vi "Neighbor.vi"(7 "Goal":T1, 10 "Dir":T2, 11 "Position":T1) -> (3 "Neighbor":T1, 5 "In Bounds":bool)   [LabVIEW 2020]
uses:
  Position.ctl
  Dir.ctl
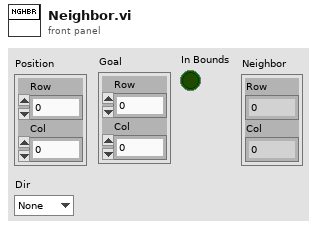
[diagram p1: front panel]
types:
  T1 = typedef "Position.ctl" = cluster{"Row":i32, "Col":i32}
  T2 = typedef "Dir.ctl" = enum16{"None", "Up", "Left", "Down", "Right"}
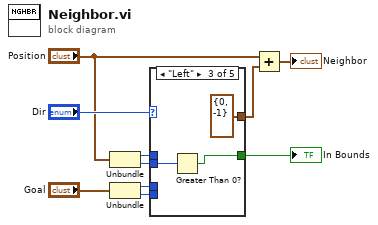
[diagram p0: block diagram]
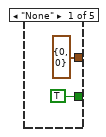
[diagram p2: hidden frame]
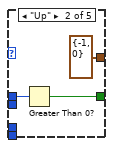
[diagram p3: hidden frame]
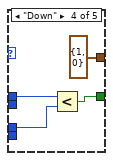
[diagram p4: hidden frame]
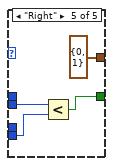
[diagram p5: hidden frame]
diagram:
  n1 = Unbundle("Position") -> ("Row"=w6:i32, "Col"=w5:i32)
  n2 = Unbundle("Goal") -> ("Row"=w2:i32, "Col"=w1:i32)
  n3 = case shown="\"Left\"" "Dir" {
    tunnel: [T1 {"Row"=0, "Col"=0} ("Position") T1 {"Row"=-1, "Col"=0} ("Position") T1 {"Row"=0, "Col"=-1} ("Position") T1 {"Row"=1, "Col"=0} ("Position") T1 {"Row"=0, "Col"=1} ("Position")] -> w8
    tunnel: w6 -> [_ w14 _ w21 _]
    tunnel: w5 -> [_ _ w17 _ w25]
    tunnel: [TRUE w13 w16 w19 w23] -> w4
    tunnel: w2 -> [_ _ _ w20 _]
    tunnel: w1 -> [_ _ _ _ w24]
    frame "None" {
    }
    frame "Up" {
      n4 = Greater Than 0?(x=w14) -> (x > 0?=w13:bool)
    }
    frame "Left" {
      n5 = Greater Than 0?(x=w17) -> (x > 0?=w16:bool)
    }
    frame "Down" {
      n6 = Less?(x=w21, y=w20) -> (x < y?=w19:bool)
    }
    frame "Right" {
      n7 = Less?(x=w25, y=w24) -> (x < y?=w23:bool)
    }
  }
  "In Bounds" <- w4
  n8 = Add(x="Position", y=w8) -> (x+y=→"Neighbor":T1)
